vi "Get Output Polarity.vi"(8 "error in (no error)":errorcluster {"code" format="%.0x"}, 9 "RearTriggerNo":i32=1 format="%.0g", 11 "instrument handle":refnum<k15>) -> (0 "error out":errorcluster {"code" format="%.0x"}, 2 "RetVal":i32, 3 "instrument handle out":refnum<k15>)   [LabVIEW 2021, in "Keysight XSAnVMA.lvlib"]
doc: "Returns the output to the Trigger 1 Out connector to trigger on either the positive or negative polarity."
uses:
  <instrlib>/Keysight XSAnVMA/Keysight XSAnVMA.lvlib
  KtXSAnVMA_64.dll
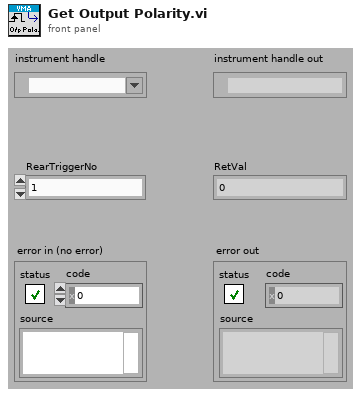
[diagram p1: front panel]
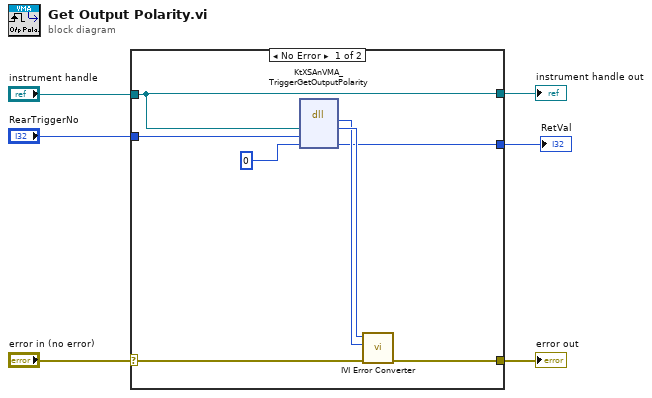
[diagram p0: block diagram]
diagram:
  n1 = case shown="No Error" "error in (no error)" {
    selector: "error in (no error)" -> [w12 w16]
    tunnel: [w11 w16] -> w6
    tunnel: "instrument handle" -> [w7 w15]
    tunnel: "RearTriggerNo" -> [w10 _]
    tunnel: [w8 _] -> w2
    tunnel: [w7 w15] -> w1
    frame No Error {
      n2 = dll-call lib="KtXSAnVMA**.dll" fn="KtXSAnVMA_TriggerGetOutputPolarity"("Vi"=w7, "RearTriggerNo"=w10, "RetVal"=0) -> (w13:i32, "Vi"=w14:u32, "RetVal"=w8:i32)  [unwired: 4 in, 2 out]
      n3 = call <instrlib>:"IVI Error Converter.vi"("error in (no error)"=w12, "IVI error code (0)"=w13, "instrument handle"=w14) -> ("error out"=w11:errorcluster)  [unwired: 7 in, 1 out]
    }
    frame Error {
    }
  }
  "error out" <- w6
  "instrument handle out" <- w1
  "RetVal" <- w2
